vi "MES_SN&WO.vi"(7 "消息框":refnum<vi>, 8 "错误输入（无错误）":errorcluster, 10 "sn":string, 11 "wo":string) -> (0 "错误输出":errorcluster, 1 "Message":string, 2 "KPSN_OK":bool)   [LabVIEW 2015]
uses:
  Global.vi
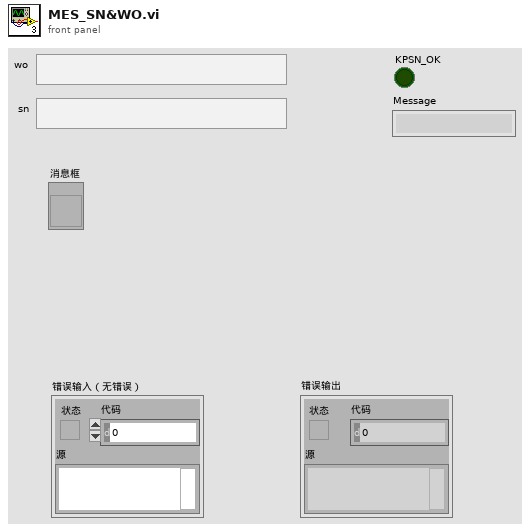
[diagram p1: front panel]
types:
  T1 = cluster{"URL":string, "audit_mode":string, "tsid":string, "model":string, "product":string, "test_station":string, "station_id":string, "test_station_name":string, "Webservice":string}
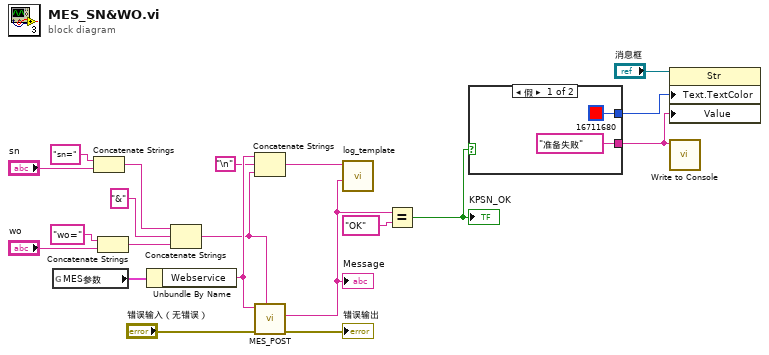
[diagram p0: block diagram]
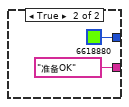
[diagram p2: hidden frame]
diagram:
  n1 = global read "Global.vi" "MES参数"() -> (w20:T1)
  n2 = Concatenate Strings("sn=", "sn") -> (w17:string)
  n3 = Concatenate Strings("wo=", "wo") -> (w14:string)
  n4 = Unbundle By Name(w20) -> ("Webservice"=w9:string)
  n5 = Concatenate Strings(w17, "&", w14) -> (w7:string)
  n6 = Concatenate Strings(w9, "\n", w7) -> (w6:string)
  n7 = call "MES_POST.vi"("DATA"=w7, "错误输入（无错误）"="错误输入（无错误）", "URL"=w9) -> ("错误输出"=→"错误输出":errorcluster, "body"=w1:string)  [unwired: 6 in, 1 out]
  "Message" <- w1
  n8 = call "log_template.vi"("接收报文"=w1, "发送报文"=w6) -> ()  [unwired: 10 in]
  n9 = Equal?(x=w1, y="OK") -> (x = y?=w4:bool)
  "KPSN_OK" <- w4
  n10 = case shown="假" w4 {
    tunnel: ["准备失败" "准备OK"] -> w2
    tunnel: [u32 16711680 u32 6618880] -> w3
    frame False {
    }
    frame True {
    }
  }
  n11 = property class="Str"(reference="消息框", "Text.TextColor"=w3, "Value"=w2) -> ()  [unwired: 1 in, 2 out]
  n12 = call "Write to Console.vi"("Input"=w2) -> ()  [unwired: 10 in, 1 out]
